vi "Test_Dataq_ReadAIn.vi"(8 "error in (no error)":errorcluster, 10 "Num Chan":i32=2, 11 "VISA Refnum in":refnum<visa-resource-name>="COM3") -> (0 "error out":errorcluster={"status"=FALSE, "code"=1073676294, "source"="VISA Read in IO_Dataq_ReadAIn.vi->_OLS_Main.vi"}, 1 "Outputs":dbl[](array[numeric]), 2 "Waveform Chart":dbl[][](graph), 3 "VISA Refnum out":refnum<visa-resource-name>="COM3", 4 "Bytes at Port":u32=12352)   [LabVIEW 2024]
panel:
  out "Boolean":bool
  in  "stop":bool
  out "Array":dbl[][](array[numeric])
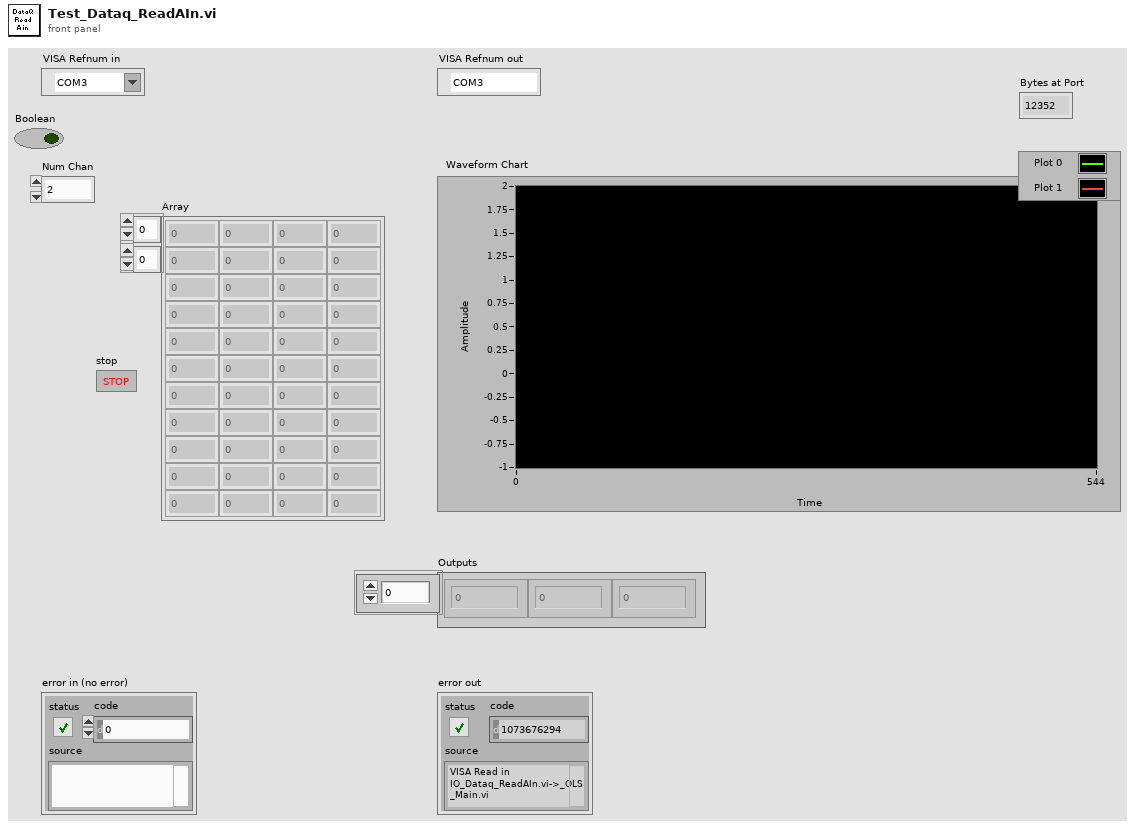
[diagram p1: front panel]
types:
  T1 = enum16{"big-endian, network order", "native, host order", "little-endian"}
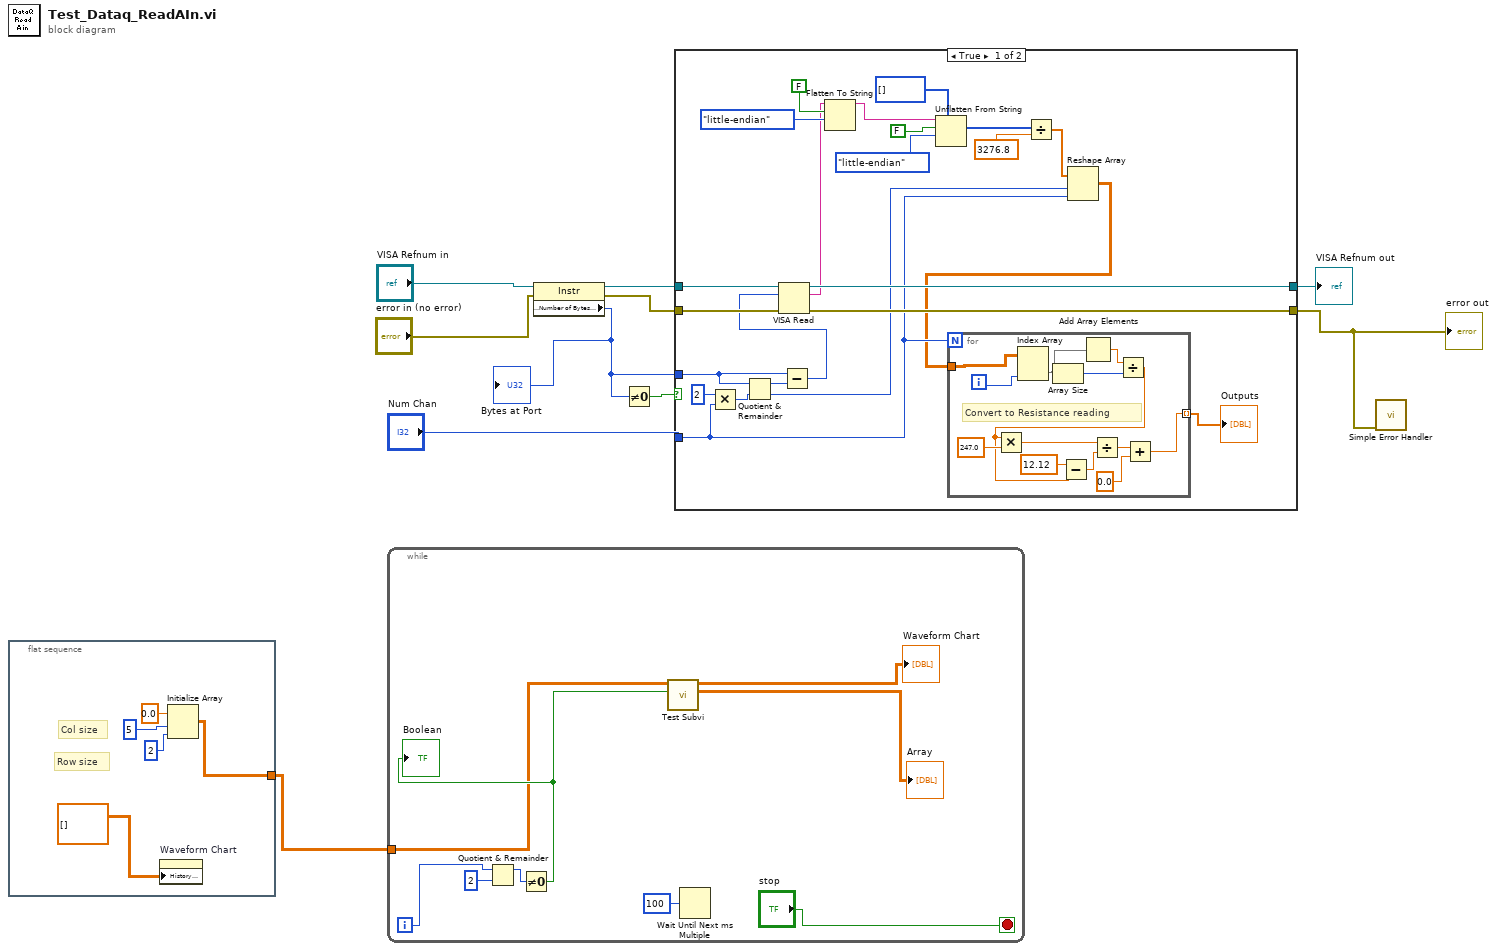
[diagram p0: block diagram]
diagram:
  n1 = flat-sequence {
    tunnel: [w12] -> w2
    frame #0 {
      # "Row size"
      # "Col size"
      n2 = property on="Waveform Chart" class="WFChart (strict)"("History Data"=dbl[][] [] ("Waveform Chart")) -> ()  [unwired: 2 in, 2 out]
      n3 = Initialize Array(0.0 ("element"), 5 ("dimension size"), 2 ("dimension size")) -> (w12:dbl[][])
    }
  }
  n4 = while {
    tunnel: w2 -> [w18]
    i -> [w20]
    stop <- "stop" stop-if-true
    n5 = Quotient & Remainder(x=w20, y=2) -> (x-y*floor(x/y)=w22:i32)  [unwired: 1 out]
    n6 = Not Equal To 0?(x=w22) -> (x != 0?=w19:bool)
    "Boolean" <- w19
    n7 = call "Test Subvi.vi"("Boolean"=w19, "Array in"=w18) -> ("Array out"=→"Array":dbl[][], "Waveform Chart"=→"Waveform Chart":dbl[][])  [unwired: 8 in]
    n8 = Wait Until Next ms Multiple(millisecond multiple=u32 100) -> ()  [unwired: 1 out]
  }
  n9 = property class="Instr"(reference="VISA Refnum in", error in="error in (no error)") -> (reference out=w5:refnum<visa-resource-name>, error out=w7:errorcluster, "Serial Settings:Number of Bytes at Serial Port"=w8:u32)
  "Bytes at Port" <- w8
  n10 = Not Equal To 0?(x=w8) -> (x != 0?=w9:bool)
  n11 = case shown="True" w9 {
    tunnel: [w46 w61] -> w3
    tunnel: w7 -> [w47 w62]
    tunnel: [w42 w62] -> w1
    tunnel: w5 -> [w29 w61]
    tunnel: w8 -> [w28 _]
    tunnel: "Num Chan" -> [w27 _]
    frame True {
      n12 = Multiply(x=2, y=w27) -> (x*y=w30:i32)
      n13 = Quotient & Remainder(x=w28, y=w30) -> (x-y*floor(x/y)=w44:u32, floor(x/y)=w32:u32)
      n14 = Subtract(x=w28, y=w44) -> (x-y=w43:u32)
      n15 = VISA Read(VISA resource name=w29, byte count=w43, error in (no error)=w47) -> (VISA resource name out=w46:refnum<visa-resource-name>, read buffer=w36:string, error out=w42:errorcluster)  [unwired: 1 out]
      n16 = Flatten To String(anything=w36, prepend array or string size? (T)=FALSE, byte order (0:big-endian, network order)=T1."little-endian") -> (data string=w37:string)  [unwired: 1 in, 2 out]
      n17 = Unflatten From String(type=i16[] [], binary string=w37, data includes array or string size? (T)=FALSE, byte order (0:big-endian, network order)=T1."little-endian") -> (value=w35:i16[])  [unwired: 1 in, 2 out]
      n18 = Divide(x=w35, y=3276.8) -> (x/y=w33:dbl[])
      n19 = Reshape Array(w33, w32, w27) -> (w26:dbl[][])
      n20 = for {
        N: w27 -> [_]
        tunnel: w26 -> [w60]
        tunnel: [w48] -> w25 mode=indexing
        i -> [w56]
        # "Convert to Resistance reading"
        n21 = Index Array(array=w60, index (col)=w56) -> (element=w57:dbl[])  [unwired: 1 in]
        n22 = Array Size(array=w57) -> (size(s)=w58:i32)
        n23 = Add Array Elements(numeric array=w57) -> (sum=w59:dbl)
        n24 = Divide(x=w59, y=w58) -> (x/y=w53:dbl)
        n25 = Multiply(x=w53, y=247.0) -> (x*y=w51:dbl)
        n26 = Subtract(x=12.12, y=w53) -> (x-y=w52:dbl)
        n27 = Divide(x=w51, y=w52) -> (x/y=w50:dbl)
        n28 = Add(x=w50, y=0.0) -> (x+y=w48:dbl)
      }
      "Outputs" <- w25
    }
    frame False {
    }
  }
  "error out" <- w1
  "VISA Refnum out" <- w3
  n29 = call <vilib>:"Simple Error Handler.vi"("error in (no error)"=w1) -> ()  [unwired: 4 in, 5 out]
